vi "Segment Shape.vi"(5 "edgetime (0.2)":dbl=0.2, 7 "downtime (0.1)":dbl=0.1, 11 "x (0..1)":dbl) -> (3 "y (0..1)":dbl)   [LabVIEW 2025]
doc: "Generates a curve with a devined downtime, rise time and hightime over an interval of x = 0..1"
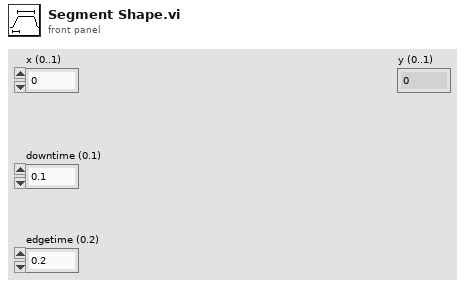
[diagram p1: front panel]
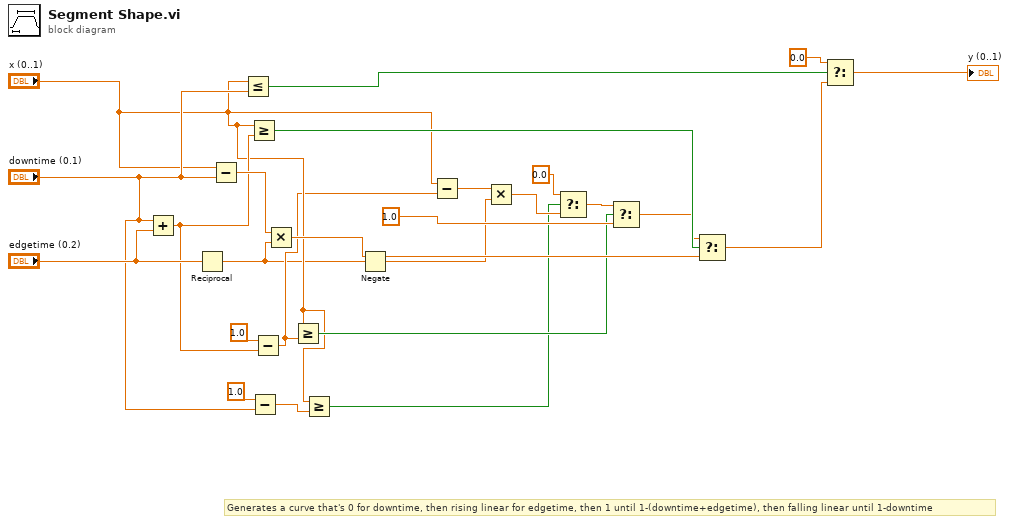
[diagram p0: block diagram]
diagram:
  # "Generates a curve that's 0 for downtime, then rising linear for edgetime, then 1 until 1-(downtime+edgetime), then falling linear until 1-downtime"
  n1 = Add(x="downtime (0.1)", y="edgetime (0.2)") -> (x+y=w15:dbl)
  n2 = Reciprocal(x="edgetime (0.2)") -> (1/x=w6:dbl)
  n3 = Subtract(x="x (0..1)", y="downtime (0.1)") -> (x-y=w22:dbl)
  n4 = Less Or Equal?(x="x (0..1)", y="downtime (0.1)") -> (x <= y?=w25:bool)
  n5 = Greater Or Equal?(x="x (0..1)", y=w15) -> (x >= y?=w18:bool)
  n6 = Subtract(x=1.0, y="downtime (0.1)") -> (x-y=w12:dbl)
  n7 = Subtract(x=1.0, y=w15) -> (x-y=w8:dbl)
  n8 = Multiply(x=w22, y=w6) -> (x*y=w21:dbl)
  n9 = Greater Or Equal?(x="x (0..1)", y=w8) -> (x >= y?=w10:bool)
  n10 = Greater Or Equal?(x="x (0..1)", y=w12) -> (x >= y?=w2:bool)
  n11 = Negate(x=w6) -> (-x=w5:dbl)
  n12 = Subtract(x="x (0..1)", y=w8) -> (x-y=w7:dbl)
  n13 = Multiply(x=w7, y=w5) -> (x*y=w4:dbl)
  n14 = Select(t=0.0, s=w2, f=w4) -> (s? t:f=w3:dbl)
  n15 = Select(t=w3, s=w10, f=1.0 ("t")) -> (s? t:f=w11:dbl)
  n16 = Select(t=w11, s=w18, f=w21) -> (s? t:f=w19:dbl)
  n17 = Select(t=0.0, s=w25, f=w19) -> (s? t:f=→"y (0..1)":dbl)
